vi "Configure System Dialog.vi"(8 "error in (no error)":errorcluster, 11 "System Configuration In":T2={"Name"="Chamber1", "Description"="", "Logging Computer Name"="", "Logging Database Name"="", "Logging Database Path"=path "", "Archive Computer Name"="", "Archive Database Name"="", "Archive Database Path"=path "", "Lifespan (days)"=0, "Archive Enabled"=FALSE, "Archive Interval (hours)"=0, "Subsystems"=[]}) -> (0 "error out":errorcluster, 2 "Changed?":bool, 3 "System Configuration Out":T2={"Name"="Chamber1", "Description"="", "Logging Computer Name"="", "Logging Database Name"="", "Logging Database Path"=path "", "Archive Computer Name"="", "Archive Database Name"="", "Archive Database Path"=path "", "Lifespan (days)"=0, "Archive Enabled"=FALSE, "Archive Interval (hours)"=0, "Subsystems"=[]}, 4 "Subsystems Added":T1[](array[typedef]), 6 "Subsystems Deleted":T1[](array[typedef]))   [LabVIEW 2024]
doc: "This VI is a user interface VI and is used to configure the system."
uses:
  Controls/Server/System Configuration.ctl
  Controls/Server/Subsystem Configuration.ctl
panel:
  in  "Lifespan (days)":u32
  in  "Show Subsystem I/O Attributes Dialog":bool
  in  "Remove Subsystem":bool
  in  "Add Subsystem":bool
  in  "Subsystems":i32(listbox)
  in  "Logging Database Path":path
  in  "Description":string
  in  "System Name":string
  in  "Database Name":string
  in  "Computer":string
  in  "Cancel":bool
  in  "OK":bool
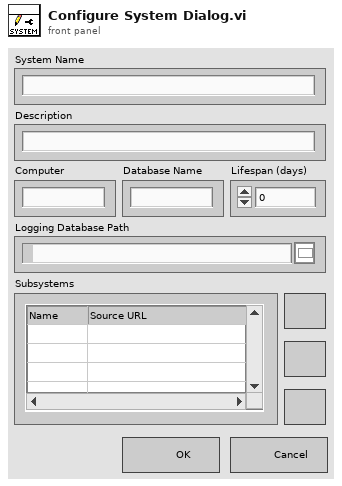
[diagram p1: front panel]
types:
  T1 = typedef "Subsystem Configuration.ctl" = cluster{"Name":string, "Root URL":refnum<k21>}
  T2 = typedef "System Configuration.ctl" = cluster{"Name":string, "Description":string, "Logging Computer Name":string, "Logging Database Name":string, "Logging Database Path":path, "Archive Computer Name":string, "Archive Database Name":string, "Archive Database Path":path, "Lifespan (days)":u32, "Archive Enabled":bool, "Archive Interval (hours)":u32, "Subsystems":T1[]}
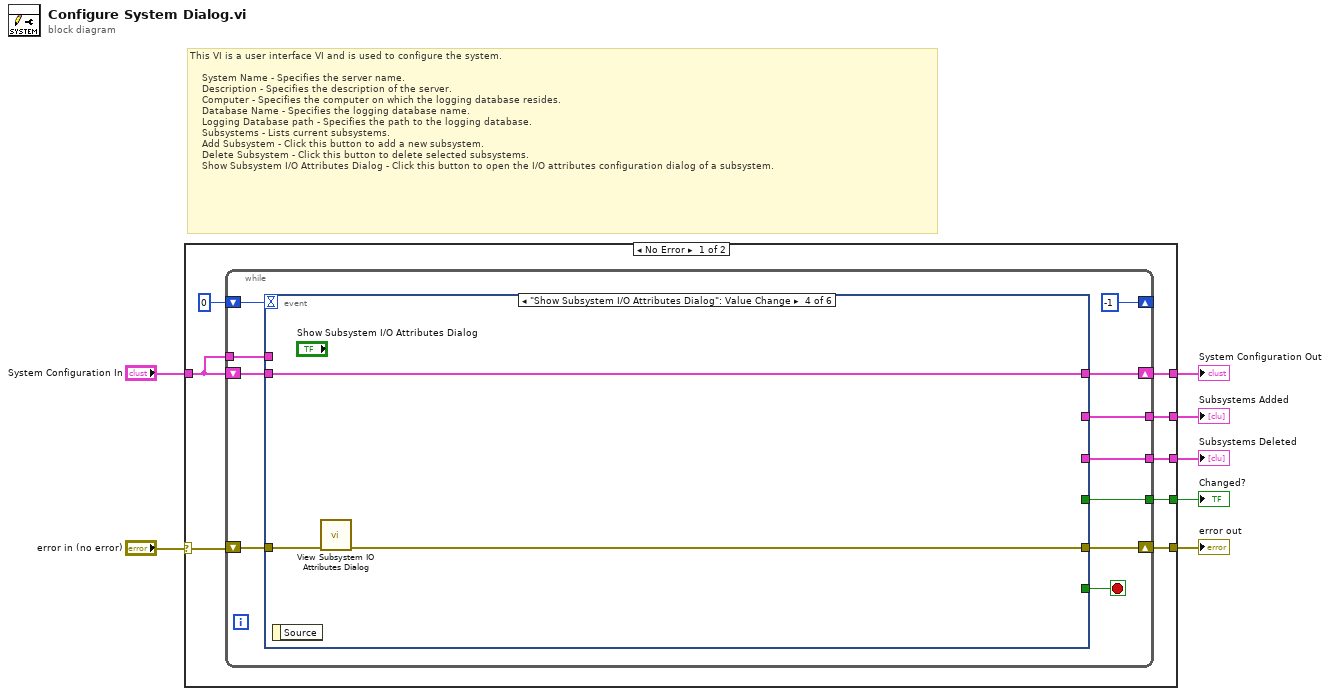
[diagram p0: block diagram]
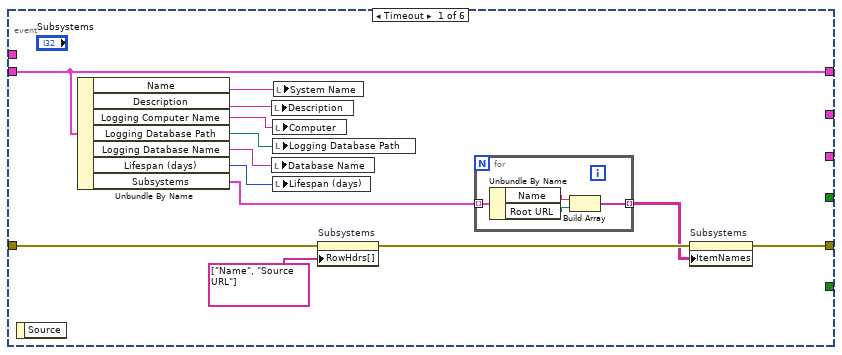
[diagram p2: hidden frame]
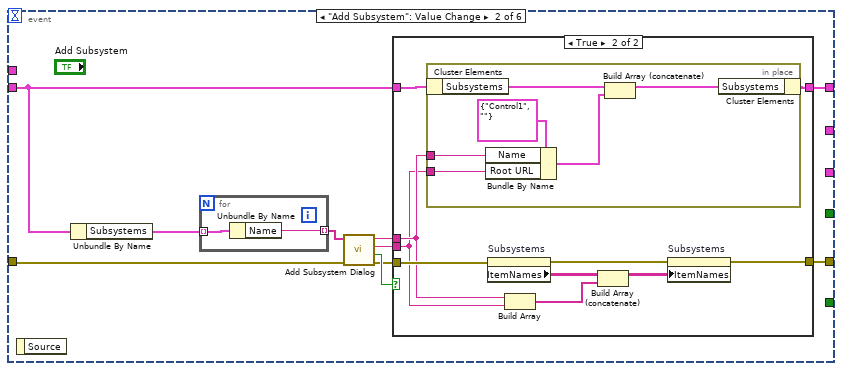
[diagram p3: hidden frame]
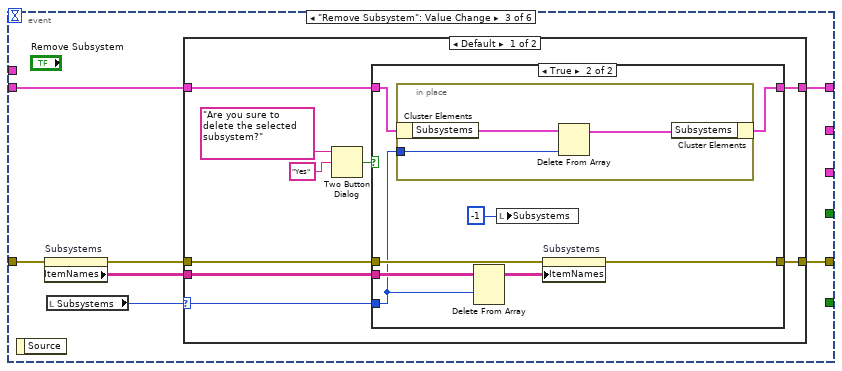
[diagram p5: hidden frame]
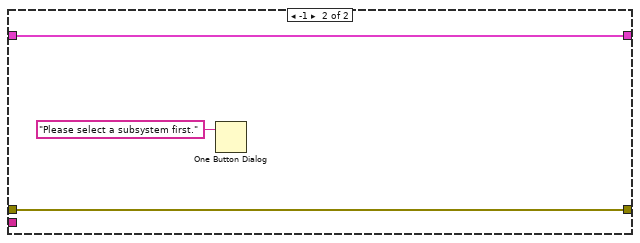
[diagram p7: hidden frame]
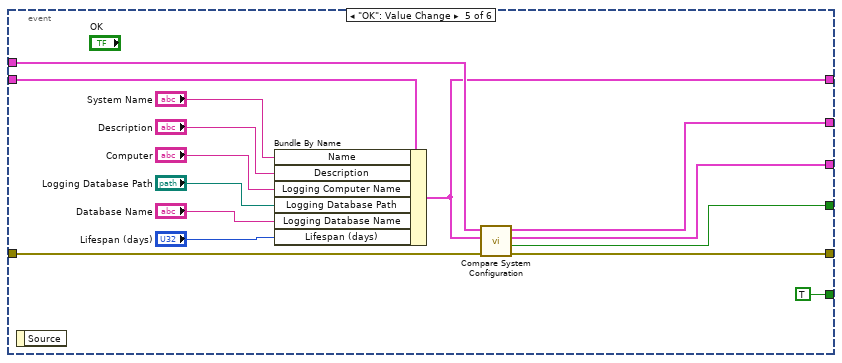
[diagram p8: hidden frame]
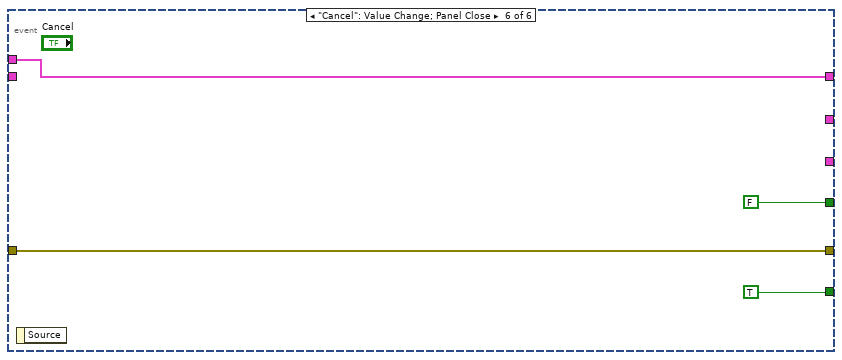
[diagram p9: hidden frame]
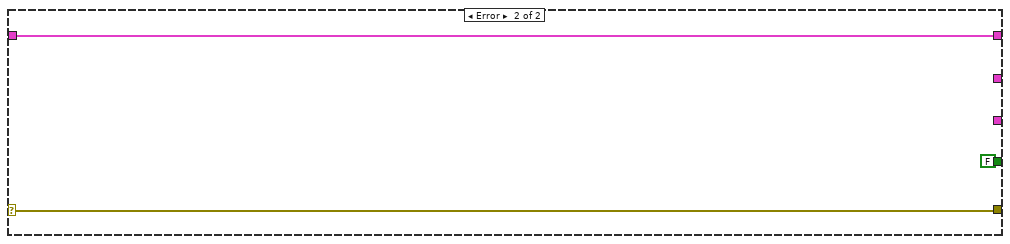
[diagram p10: hidden frame]
diagram:
  # "This VI is a user interface VI and is used to configure the system.\n\n    System Name - Specifies the server name.\n    Description - Specifies the description of the server.\n    Computer - Specifies the computer on which the logging database resides.\n    Database Name - Specifies the logging database name.\n    Logging Database path - Specifies the path to the logging database.\n    Subsystems - Lists current subsystems.\n    Add Subsystem - Click this button to add a new subsystem.\n    Delete Subsystem - Click this button to delete selected subsystems.\n    Show Subsystem I/O Attributes Dialog - Click this button to open the I/O attributes configuration dialog of a subsystem."
  n1 = case shown="No Error" "error in (no error)" {
    selector: "error in (no error)" -> [w11 w130]
    tunnel: [w8 w130] -> w6
    tunnel: "System Configuration In" -> [w12 w129]
    tunnel: [w15 w129] -> w4
    tunnel: [w14 FALSE ("UI Refresh Needed?")] -> w3
    tunnel: [w10 _] -> w2
    tunnel: [w9 _] -> w1
    frame No Error {
      n2 = while {
        shift-right: [w25] -> w15
        shift-left: w12 -> [w26]
        shift-right: [w21] -> w8
        shift-left: w11 -> [w22]
        tunnel: w12 -> [w23]
        tunnel: [w20] -> w14
        shift-right: [-1] -> _
        shift-left: 0 -> [w19]
        tunnel: [w18] -> w10
        tunnel: [w17] -> w9
        stop <- w24 stop-if-true
        n3 = event shown="[3] \"Show Subsystem I/O Attributes Dialog\": Value Change" {
          selector: _ -> [_ _ _ _ _ _]
          dyn-events: _ -> [_ _ _ _ _ _]
          timeout: w19 -> [_ _ _ _ _ _]
          tunnel: w26 -> [w39 w45 w78 w108 w117 _]
          tunnel: [w39 w53 w77 w108 w112 w124] -> w25
          tunnel: [_ _ _ _ TRUE TRUE] -> w24
          tunnel: w23 -> [_ _ _ _ w113 w124]
          tunnel: w22 -> [w38 w46 w79 w107 w115 w126]
          tunnel: [w28 w52 w75 w106 w114 w126] -> w21
          tunnel: [_ _ _ _ w109 FALSE ("UI Refresh Needed?")] -> w20
          tunnel: [_ _ _ _ w111 _] -> w18
          tunnel: [_ _ _ _ w110 _] -> w17
          event Timeout {
            n4 = event-data() -> ()  [unwired: 1 in, 1 out]
            n5 = Unbundle By Name(w39) -> ("Name"=w37:string, "Description"=w36:string, "Logging Computer Name"=w33:string, "Logging Database Path"=w35:path, "Logging Database Name"=w34:string, "Lifespan (days)"=w29:u32, "Subsystems"=w32:T1[])
            n6 = local write "Description"(w36) -> ()
            n7 = local write "Database Name"(w34) -> ()
            n8 = local write "Computer"(w33) -> ()
            n9 = local write "Logging Database Path"(w35) -> ()
            n10 = local write "Lifespan (days)"(w29) -> ()
            n11 = local write "System Name"(w37) -> ()
            n12 = property on="Subsystems" class="MCListbox (strict)"(error in=w38, "RowHdrs[]"=string[] ["Name", "Source URL"] ("Row Header Strings[]")) -> (error out=w30:errorcluster)  [unwired: 1 in, 1 out]
            n13 = for {
              tunnel: w32 -> [w43] mode=indexing
              tunnel: [w40] -> w27 mode=indexing
              n14 = Unbundle By Name(w43) -> ("Name"=w42:string, "Root URL"=w41:refnum<k21>)
              n15 = Build Array(w42, w41) -> (w40:string[])
            }
            n16 = property on="Subsystems" class="MCListbox (strict)"(error in=w30, "ItemNames"=w27) -> (error out=w28:errorcluster)  [unwired: 1 in, 1 out]
          }
          event "Add Subsystem": Value Change {
            n17 = event-data() -> ()  [unwired: 1 in, 1 out]
            n18 = Unbundle By Name(w45) -> ("Subsystems"=w48:T1[])
            n19 = for {
              tunnel: w48 -> [w55] mode=indexing
              tunnel: [w54] -> w44 mode=indexing
              n20 = Unbundle By Name(w55) -> ("Name"=w54:string)
            }
            n21 = call "Add Subsystem Dialog.vi"("error in (no error)"=w46, "Existing Subsystems"=w44) -> ("error out"=w47:errorcluster, "OK?"=w49:bool, "URL Out"=w50:string, "Subsystem Name Out"=w51:string)  [unwired: 6 in]
            n22 = case shown="True" w49 {
              tunnel: w45 -> [w57 w64]
              tunnel: [w57 w63] -> w53
              tunnel: [w56 w67] -> w52
              tunnel: w51 -> [_ w62]
              tunnel: w47 -> [w56 w66]
              tunnel: w50 -> [_ w61]
              frame False {
              }
              frame True {
                n23 = in-place {
                  in-place-border: w62 -> [w72]
                  in-place-border: w61 -> [w71]
                  n24 = in-place-cluster #1(w64) -> ("Subsystems"=w70:T1[])
                  n25 = Bundle By Name(cluster=T1 {"Name"="Control1", "Root URL"=""} ("new element/subarray"), "Name"=w72, "Root URL"=w71) -> (w68:T1)
                  n26 = Build Array (concatenate)(w70, w68) -> (w69:T1[])
                  n27 = in-place-cluster #1("Subsystems"=w69) -> (w63:T2)
                }
                n28 = property on="Subsystems" class="MCListbox (strict)"(error in=w66) -> (error out=w65:errorcluster, "ItemNames"=w60:string[][])  [unwired: 1 in, 1 out]
                n29 = Build Array(w62, w61) -> (w58:string[])
                n30 = Build Array (concatenate)(w60, w58) -> (w59:string[][])
                n31 = property on="Subsystems" class="MCListbox (strict)"(error in=w65, "ItemNames"=w59) -> (error out=w67:errorcluster)  [unwired: 1 in, 1 out]
              }
            }
          }
          event "Remove Subsystem": Value Change {
            n32 = event-data() -> ()  [unwired: 1 in, 1 out]
            n33 = property on="Subsystems" class="MCListbox (strict)"(error in=w79) -> (error out=w76:errorcluster, "ItemNames"=w80:string[][])  [unwired: 1 in, 1 out]
            n34 = local read "Subsystems"() -> (w74:i32)
            n35 = case shown="Default" w74 {
              selector: w74 -> [w85 _]
              tunnel: w80 -> [w86 _]
              tunnel: w78 -> [w84 w104]
              tunnel: [w83 w104] -> w77
              tunnel: w76 -> [w82 w103]
              tunnel: [w81 w103] -> w75
              frame Default {
                n36 = Two Button Dialog(message="Are you sure to delete the selected subsystem?", 2:"Yes" ("T button name (\"OK\")")) -> (T button?=w87:bool)  [unwired: 1 in]
                n37 = case shown="True" w87 {
                  tunnel: w86 -> [_ w96]
                  tunnel: w85 -> [_ w92]
                  tunnel: w84 -> [w90 w94]
                  tunnel: [w90 w93] -> w83
                  tunnel: w82 -> [w91 w99]
                  tunnel: [w91 w98] -> w81
                  frame False {
                  }
                  frame True {
                    n38 = in-place {
                      in-place-border: w92 -> [w100]
                      n39 = in-place-cluster #2(w94) -> ("Subsystems"=w102:T1[])
                      n40 = Delete From Array(array=w102, index=w100) -> (array with subset deleted=w101:T1[])  [unwired: 1 in, 1 out]
                      n41 = in-place-cluster #2("Subsystems"=w101) -> (w93:T2)
                    }
                    n42 = Delete From Array(array=w96, index (row)=w92) -> (array with subset deleted=w97:string[][])  [unwired: 2 in, 1 out]
                    n43 = local write "Subsystems"(-1 ("Value")) -> ()
                    n44 = property on="Subsystems" class="MCListbox (strict)"(error in=w99, "ItemNames"=w97) -> (error out=w98:errorcluster)  [unwired: 1 in, 1 out]
                  }
                }
              }
              frame -1 {
                n45 = One Button Dialog(message="Please select a subsystem first.") -> ()  [unwired: 1 in, 1 out]
              }
            }
          }
          event "Show Subsystem I/O Attributes Dialog": Value Change {
            n46 = event-data() -> ()  [unwired: 1 in, 1 out]
            n47 = call "View Subsystem IO Attributes Dialog.vi"("error in (no error)"=w107) -> ("error out"=w106:errorcluster)  [unwired: 10 in]
          }
          event "OK": Value Change {
            n48 = event-data() -> ()  [unwired: 1 in, 1 out]
            n49 = Bundle By Name(cluster=w117, "Name"="System Name", "Description"="Description", "Logging Computer Name"="Computer", "Logging Database Path"="Logging Database Path", "Logging Database Name"="Database Name", "Lifespan (days)"="Lifespan (days)") -> (w112:T2)
            n50 = call "Compare System Configuration.vi"("error in (no error)"=w115, "New System Configuration"=w112, "System Configuration"=w113) -> ("error out"=w114:errorcluster, "Changed?"=w109:bool, "Subsystems Deleted"=w110:T1[], "Subsystems Added"=w111:T1[])  [unwired: 5 in]
          }
          event "Cancel": Value Change; Panel Close {
            n51 = event-data() -> ()  [unwired: 1 in, 1 out]
          }
        }
      }
    }
    frame Error {
    }
  }
  "System Configuration Out" <- w4
  "error out" <- w6
  "Changed?" <- w3
  "Subsystems Added" <- w2
  "Subsystems Deleted" <- w1
